vi "Get ControlRef from ClassItem.vi"(8 "error in (no error)":errorcluster, 10 "Item Name":string, 11 "LVClassLibrary in":refnum<vi>) -> (0 "error out":errorcluster, 1 "Found ?":bool, 2 "Control ref out":refnum<vi>, 3 "LVClassLibrary out":refnum<vi>)   [LabVIEW 2019, in "gRPC Scripting Tools.lvlib"]
uses:
  gRPC Scripting Tools.lvlib
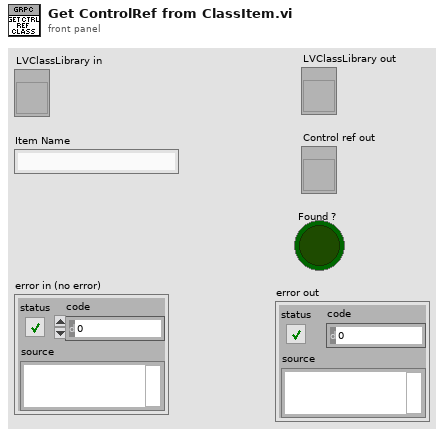
[diagram p1: front panel]
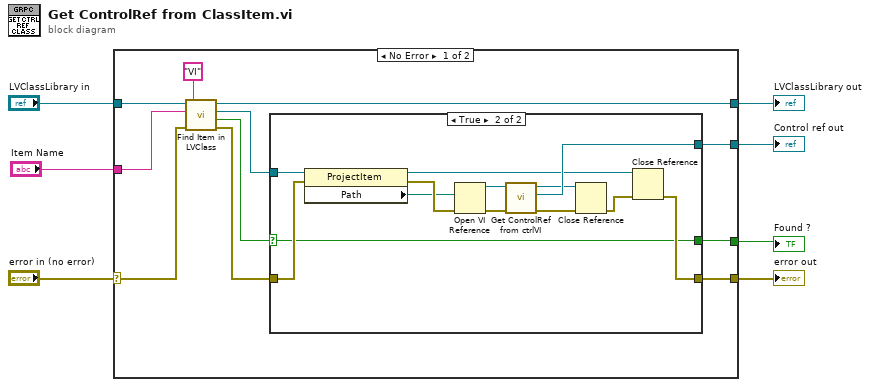
[diagram p0: block diagram]
diagram:
  n1 = case shown="No Error" "error in (no error)" {
    selector: "error in (no error)" -> [w10 w34]
    tunnel: [w18 _] -> w7
    tunnel: "LVClassLibrary in" -> [w15 w35]
    tunnel: "Item Name" -> [w13 _]
    tunnel: [w12 w35] -> w4
    tunnel: [w11 w34] -> w3
    tunnel: [w8 _] -> w1
    frame No Error {
      n2 = call "Find Item in LVClass.vi"("Item Type"="VI", "error in (no error)"=w10, "Item Name"=w13, "Class Item in"=w15) -> ("error out"=w17:errorcluster, "Found?"=w9:bool, "Project Item (Class Item)"=w16:refnum<vi>, "Class Item out"=w12:refnum<vi>)  [unwired: 4 in]
      n3 = case shown="True" w9 {
        selector: w9 -> [w19 w21]
        tunnel: [_ w31] -> w18
        tunnel: w17 -> [w20 w29]
        tunnel: w16 -> [_ w28]
        tunnel: [w20 w22] -> w11
        tunnel: [w19 w21] -> w8
        frame False {
        }
        frame True {
          n4 = property class="ProjectItem"(reference=w28, error in=w29) -> (reference out=w26:refnum<vi>, error out=w32:errorcluster, "Path"=w27:path)
          n5 = Open VI Reference(vi path=w27, error in (no error)=w32) -> (vi reference=w30:refnum<vi>, error out=w33:errorcluster)  [unwired: 4 in]
          n6 = call "Get ControlRef from ctrlVI.vi"("error in (no error)"=w33, "VI ref in"=w30) -> ("error out"=w24:errorcluster, "Control ref out"=w31:refnum<vi>, "VI ref out"=w25:refnum<vi>)  [unwired: 7 in]
          n7 = Close Reference(reference=w25, error in (no error)=w24) -> (error out=w23:errorcluster)
          n8 = Close Reference(reference=w26, error in (no error)=w23) -> (error out=w22:errorcluster)
        }
      }
    }
    frame Error {
    }
  }
  "Control ref out" <- w7
  "LVClassLibrary out" <- w4
  "error out" <- w3
  "Found ?" <- w1
